vi "Get Bit (I64).vi"(10 "Bit":u8, 11 "Number":i64 format="%.0x") -> (2 "Value":bool=TRUE, 3 "Number Out":i64 format="%.0x")   [LabVIEW 2019, in "Bits.lvlib"]
doc: "Returns the bit value of the bit in the passed in number."
uses:
  Bits.lvlib
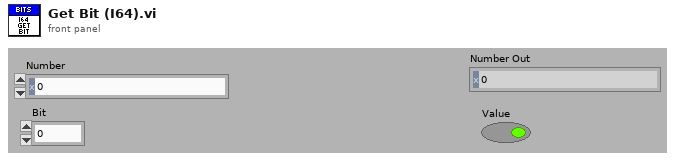
[diagram p1: front panel]
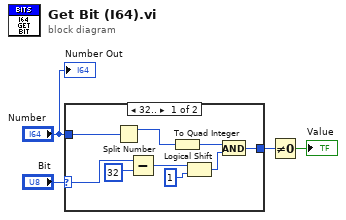
[diagram p0: block diagram]
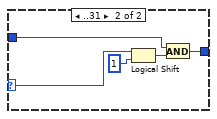
[diagram p2: hidden frame]
diagram:
  n1 = case shown="32.." "Bit" {
    selector: "Bit" -> [w11 w17]
    tunnel: "Number" -> [w9 w16]
    tunnel: [w6 w14] -> w2
    frame 32.. {
      n2 = Split Number(x=w9) -> (hi(x)=w10:u32)  [unwired: 1 out]
      n3 = Subtract(x=w11, y=u8 32 ("x")) -> (x-y=w12:u8)
      n4 = To Quad Integer(1:w10) -> (0:w5:i64)
      n5 = Logical Shift(y=w12, x=i64 1) -> (x << y=w8:i64)
      n6 = And(x=w5, y=w8) -> (x .and. y?=w6:i64)
    }
    frame ..31 {
      n7 = Logical Shift(y=w17, x=i64 1) -> (x << y=w15:i64)
      n8 = And(x=w16, y=w15) -> (x .and. y?=w14:i64)
    }
  }
  n9 = Not Equal To 0?(x=w2) -> (x != 0?=→"Value":bool)
  "Number Out" <- "Number"
